vi "Directories.vi"() -> (2 "Config.ini Path":path, 3 "Application Directory":path)   [LabVIEW 2018]
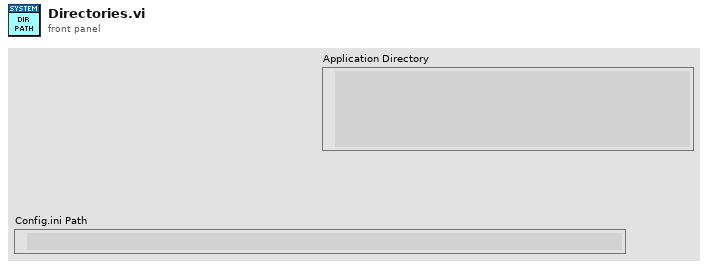
[diagram p1: front panel]
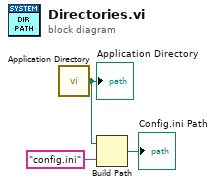
[diagram p0: block diagram]
diagram:
  n1 = call <vilib>:"Application Directory.vi"() -> ("Application Directory"=w3:path)
  "Application Directory" <- w3
  n2 = Build Path(base path=w3, name or relative path="config.ini") -> (appended path=→"Config.ini Path":path)
